vi "Structure Name To ID.vi"(8 "Error In":errorcluster, 9 "Data":string, 10 "Structure Name":string, 11 "Nest Config":T1) -> (0 "Error Out":errorcluster, 1 "Data":string, 2 "Structure ID":string, 3 "Nest Config":T1)   [LabVIEW 2013, in "LVH-Nest.lvlib"]
doc: "Get the structure ID for the specified structure name."
uses:
  LVH-Nest.lvlib
  Type Defs/Nest Config.ctl
  <vilib>/httpClient/ClientHandle.ctl
  Type Defs/Session Data.ctl
  Type Defs/Nest Error.ctl
  <vilib>/httpClient/LabVIEWHTTPClient.lvlib
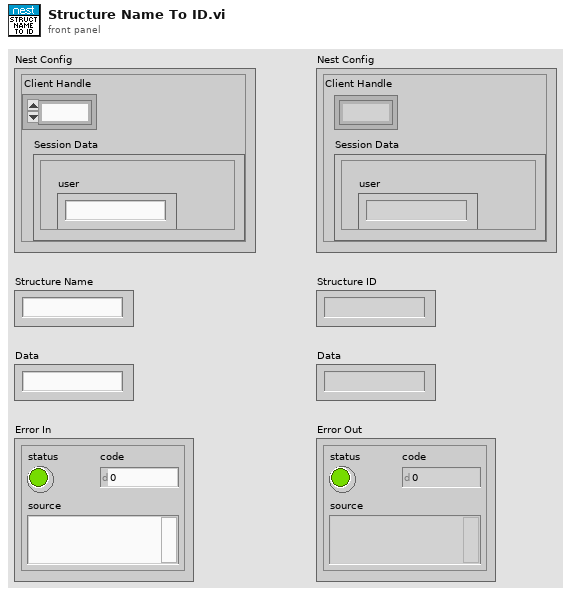
[diagram p1: front panel]
types:
  T1 = typedef "LVH-Nest.lvlib/Nest Config.ctl" = cluster{"Client Handle":T2, "Session Data":T3}
  T2 = typedef "LabVIEWHTTPClient.lvlib/ClientHandle.ctl" = refnum<k1>
  T3 = typedef "LVH-Nest.lvlib/Session Data.ctl" = cluster{"is_superuser":bool, "is_staff":bool, "urls":cluster{"transport_url":string, "rubyapi_url":string, "weather_url":string, "log_upload_url":string, "support_url":string}, "limits":cluster{"thermostats_per_structure":u32, "structures":u32, "thermostats":u32, "smoke_detectors":u32, "smoke_detectors_per_structure":u32}, "access_token":string, "userid":string, "expires_in":string, "email":string, "user":string, "language":string}
  T4 = typedef "LVH-Nest.lvlib/Nest Error.ctl" = enum16{"Unknown", "Auth", "Read", "Invalid Structure Name", "Invalid Device Name", "Set Temp"}
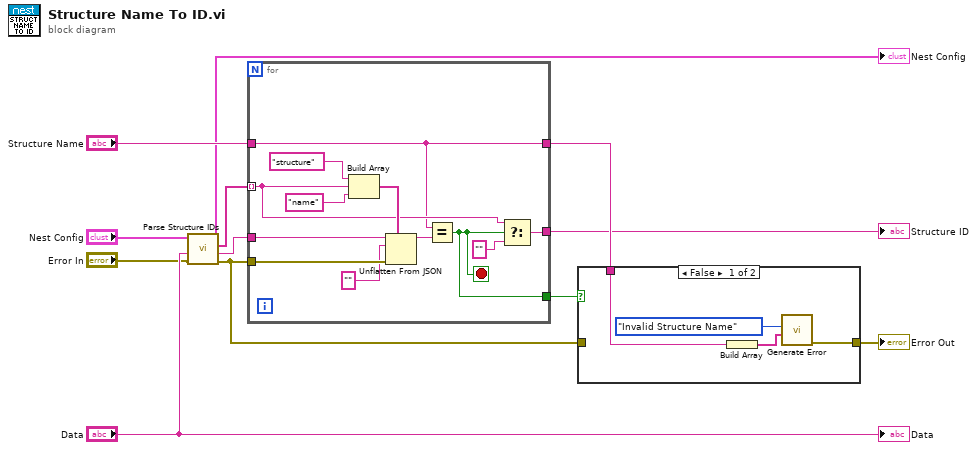
[diagram p0: block diagram]
diagram:
  n1 = call "Parse Structure IDs.vi"("Error In"="Error In", "Data"="Data", "Nest Config"="Nest Config") -> ("Error Out"=w7:errorcluster, "Data"=w5:string, "Structure IDs"=w12:string[], "Nest Config"=→"Nest Config":T1)  [unwired: 5 in]
  n2 = for {
    tunnel: w7 -> [w21]
    tunnel: w12 -> [w17] mode=indexing
    tunnel: w5 -> [w20]
    tunnel: "Structure Name" -> [w13]
    tunnel: [w15] -> w10
    tunnel: [w14] -> w4
    tunnel: [w13] -> w9
    stop <- w15 stop-if-true
    n3 = Build Array("structure", w17, "name" ("element")) -> (w22:string[])
    n4 = Unflatten From JSON(path=w22, JSON string=w20, type and defaults="" ("element"), error in (no error)=w21) -> (value=w18:string)  [unwired: 3 in, 1 out]
    n5 = Equal?(x=w13, y=w18) -> (x = y?=w15:bool)
    n6 = Select(t=w17, s=w15, f="") -> (s? t:f=w14:string)
  }
  "Structure ID" <- w4
  n7 = case shown="False" w10 {
    tunnel: [w27 w29] -> w8
    tunnel: w9 -> [w26 _]
    tunnel: w7 -> [_ w29]
    frame False {
      n8 = Build Array(w26) -> (w25:string[])
      n9 = call "Generate Error.vi"("Args"=w25, "Nest Error"=Nest_Error."Invalid Structure Name") -> ("Error Out"=w27:errorcluster)  [unwired: 9 in]
    }
    frame True {
    }
  }
  "Error Out" <- w8
  "Data" <- "Data"
